vi "CAN Database Change Manager UI.vi"(8 "error in (no error)":errorcluster, 9 "VS Existing Frames":T1[](array[typedef]) {"Node Ref" format="%.0x"}, 10 "Old Cluster":refnum<k21>) -> (0 "error out":errorcluster, 2 "Cancel Out":bool, 3 "CAN Update":T4 {"Frames to Delete" format="%.0x"; "Frames to Update"."Node Ref" format="%.0x"})   [LabVIEW 2025, in "Protection and Counter Addon System Explorer.lvlib"]
uses:
  Protection and Counter Addon System Explorer.lvlib
  Types/CAN Update Results.ctl
  <vilib>/NI VeriStand/Custom Device API/Custom Device Item Ref.ctl
  Types/CAN Frame Update Results.ctl
  Types/CAN Filter Type.ctl
  Types/Base Frame Info_NoVS.ctl
  Types/Base Frame Info.ctl
  <vilib>/Utility/cursorutil.llb/Set Cursor (Icon Pict).vi
  <resource>/objmgr/xnet.rc
  <vilib>/NI VeriStand/Custom Device API/Custom Device API.lvlib
panel:
  in  "New Cluster":u16(ring)
  in  "New Database":refnum<k21>
  in  "Export":bool
  in  "Cancel":bool
  in  "Update":bool
  in  "Tree":string(tree)
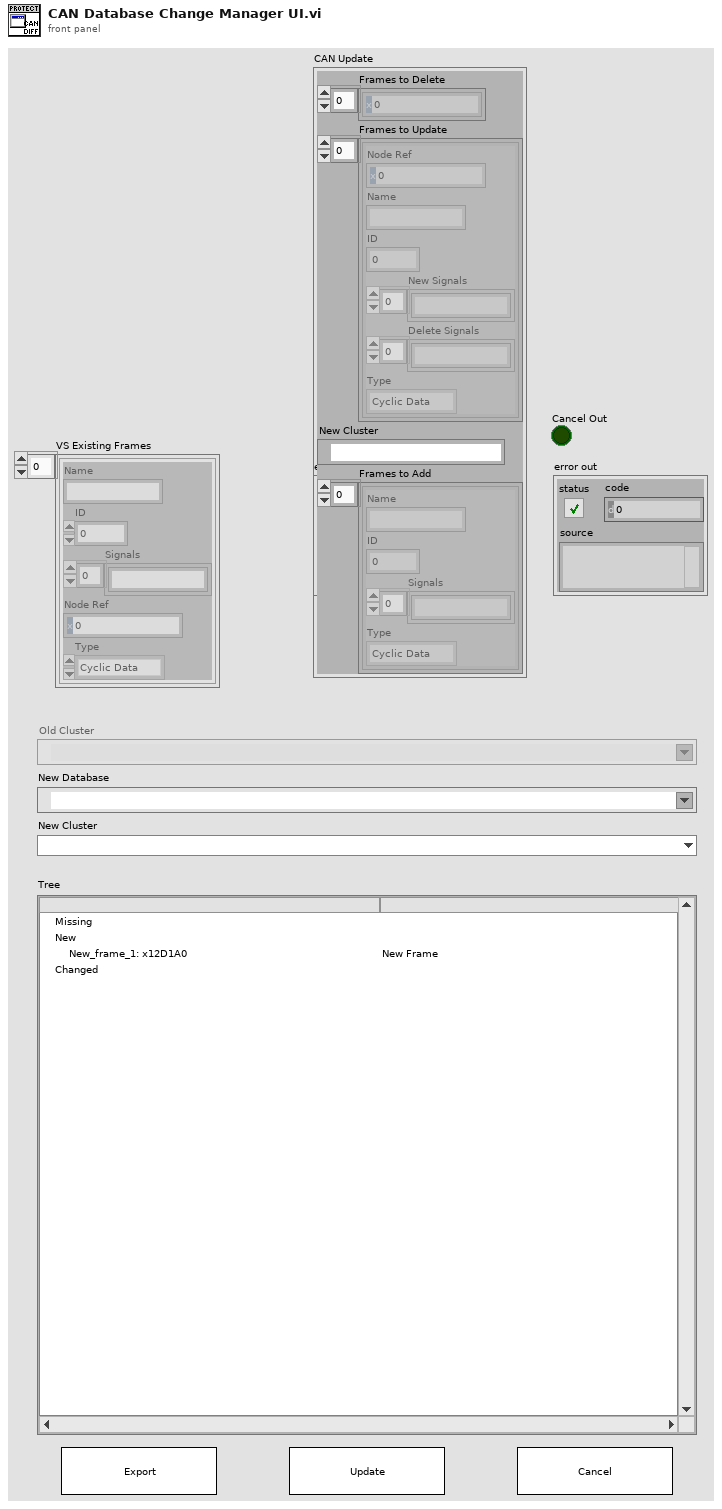
[diagram p1: front panel]
types:
  T1 = typedef "Protection and Counter Addon System Explorer.lvlib/Base Frame Info.ctl" = cluster{"Name":string, "ID":u32, "Signals":string[], "Node Ref":T2, "Type":T3}
  T2 = typedef "Custom Device API.lvlib/Custom Device Item Ref.ctl" = u64
  T3 = typedef "Protection and Counter Addon System Explorer.lvlib/CAN Filter Type.ctl" = enum16{"Cyclic Data", "Event Data", "Cyclic/Event", "All"}
  T4 = typedef "Protection and Counter Addon System Explorer.lvlib/CAN Update Results.ctl" = cluster{"Frames to Delete":T2[], "Frames to Update":T5[], "New Cluster":refnum<k21>, "Frames to Add":T6[]}
  T5 = typedef "Protection and Counter Addon System Explorer.lvlib/CAN Frame Update Results.ctl" = cluster{"Node Ref":T2, "Name":string, "ID":u32, "New Signals":string[], "Delete Signals":string[], "Type":T3}
  T6 = typedef "Protection and Counter Addon System Explorer.lvlib/Base Frame Info_NoVS.ctl" = cluster{"Name":string, "ID":u32, "Signals":string[], "Type":T3}
  T7 = enum8{"Enabled", "Disabled", "Disabled and Grayed Out"}
  T8 = typedef "Protection and Counter Addon System Explorer.lvlib/Database Changes.ctl" = cluster{"New":T6[], "Missing":T1[], "Changed":T9[]}
  T9 = typedef "Protection and Counter Addon System Explorer.lvlib/Related CAN Frames.ctl" = cluster{"Old":T1, "Change":T10}
  T10 = typedef "Protection and Counter Addon System Explorer.lvlib/Related CAN Frames No VS.ctl" = cluster{"New":T6, "Old":T6}
  T11 = typedef "LVPoint32TypeDef.ctl" = cluster{"Horizontal":i32, "Vertical":i32}
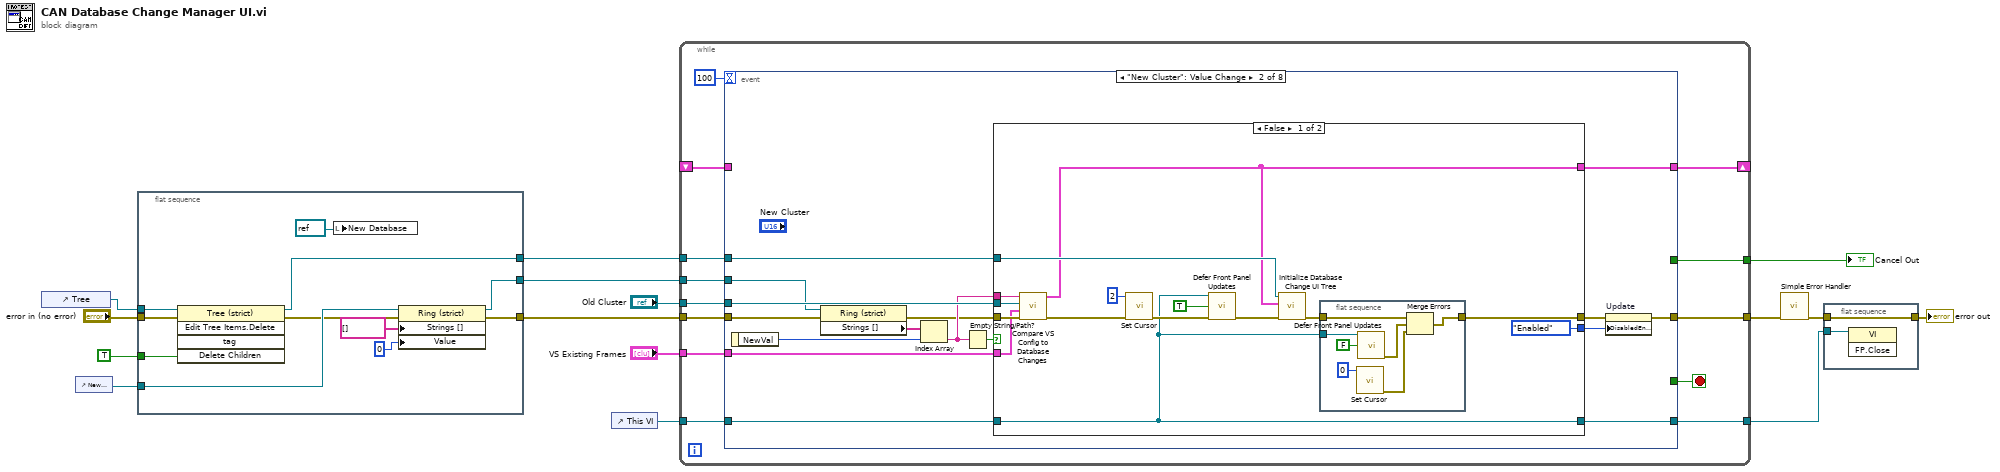
[diagram p0: block diagram]
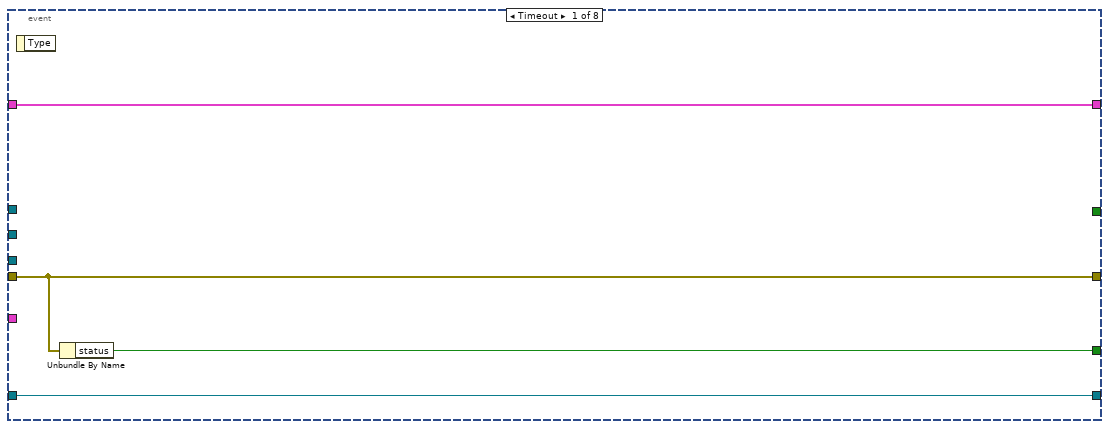
[diagram p2: hidden frame]
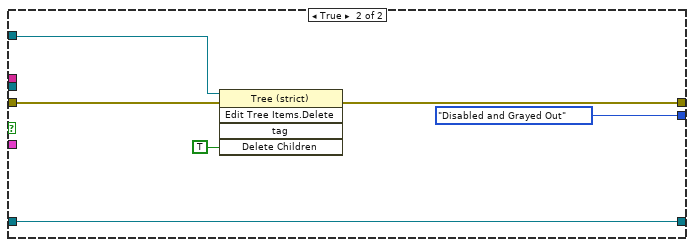
[diagram p3: hidden frame]
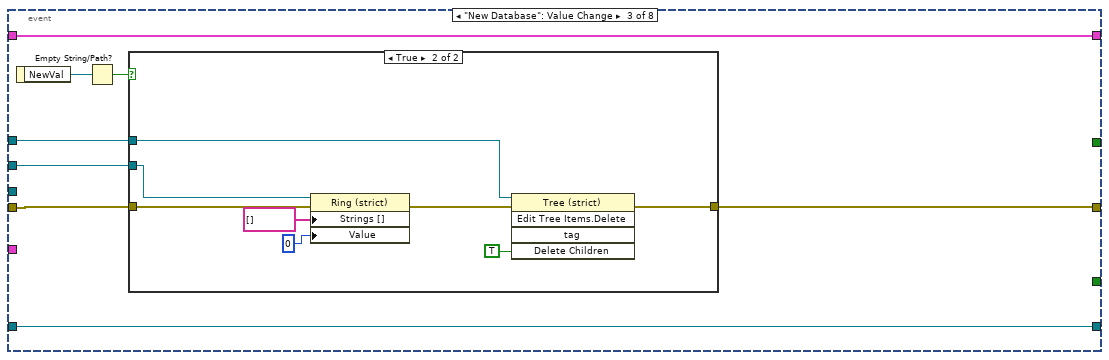
[diagram p4: hidden frame]
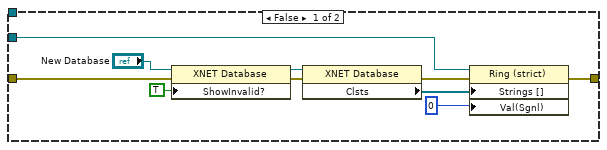
[diagram p5: hidden frame]
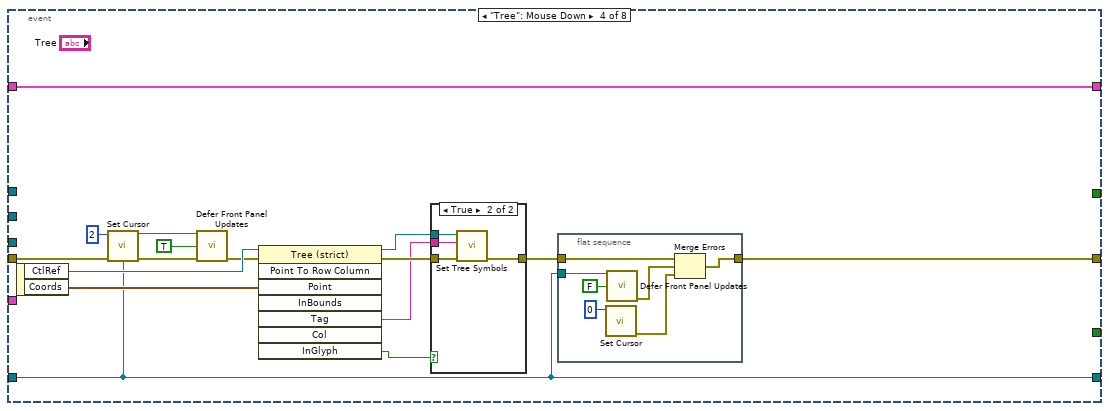
[diagram p6: hidden frame]
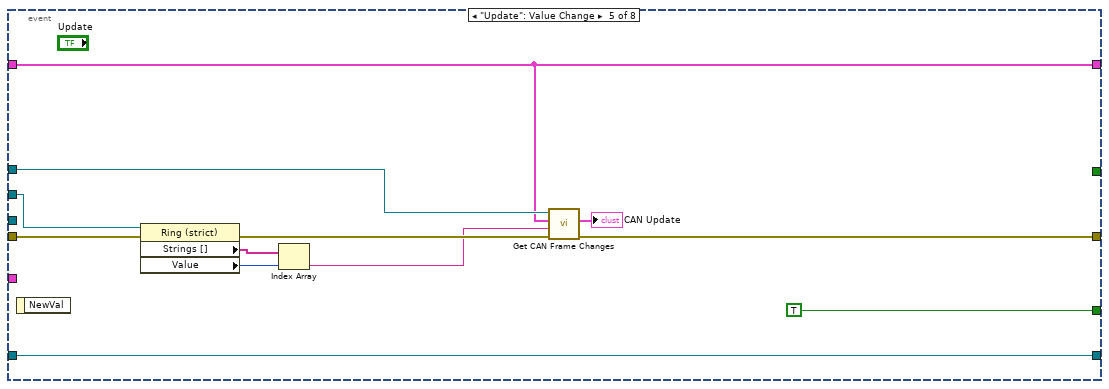
[diagram p8: hidden frame]
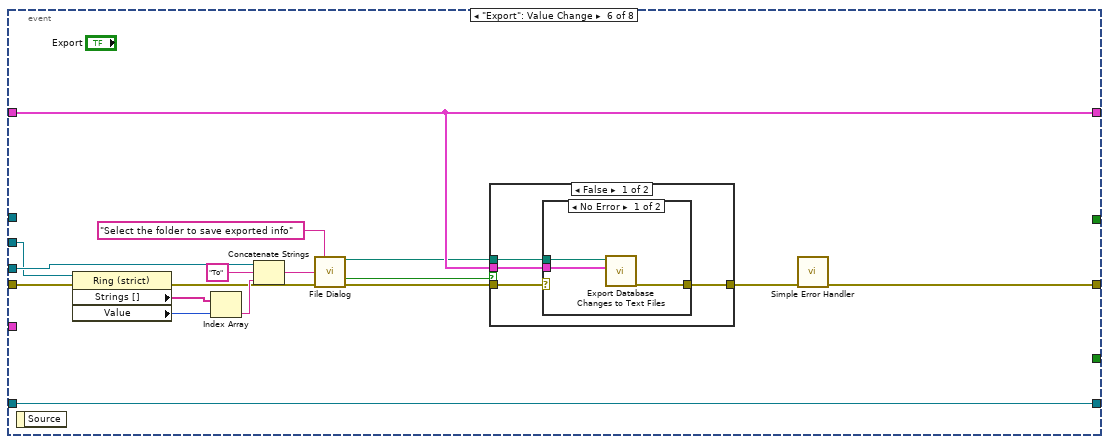
[diagram p9: hidden frame]
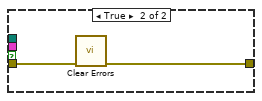
[diagram p11: hidden frame]
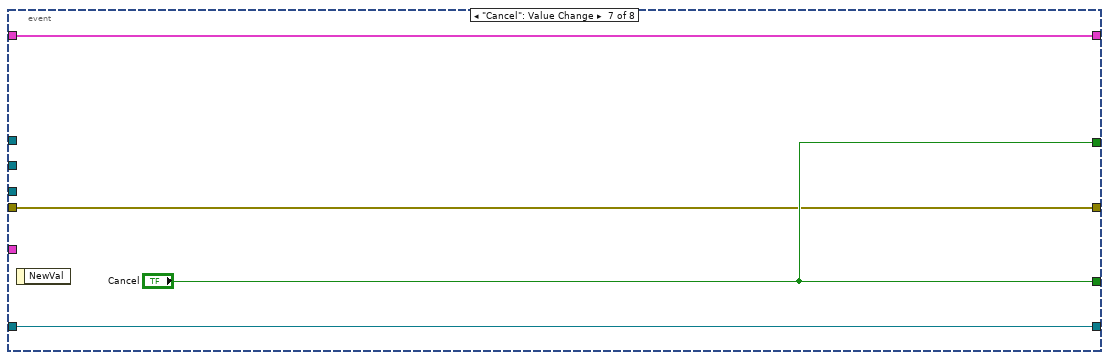
[diagram p12: hidden frame]
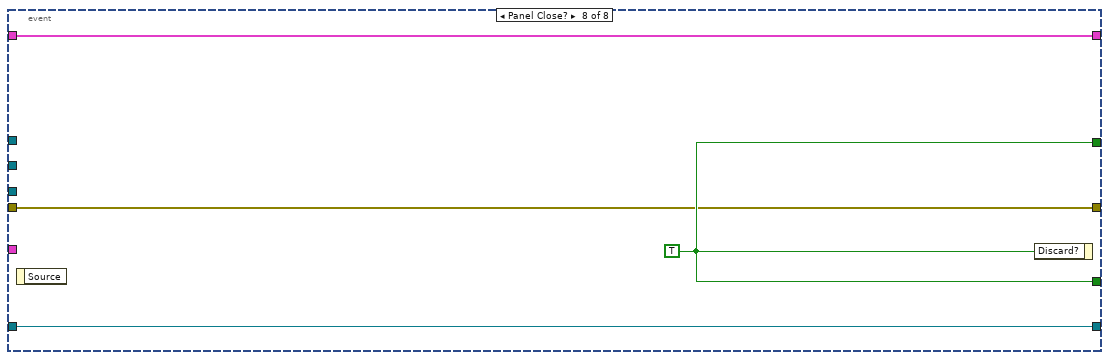
[diagram p13: hidden frame]
diagram:
  n1 = control-ref of="Tree"() -> (w6:refnum<vi>)
  n2 = control-ref of="New Cluster"() -> (w2:refnum<vi>)
  n3 = flat-sequence {
    tunnel: TRUE ("Delete Children?") -> [w26]
    tunnel: w6 -> [w25]
    tunnel: [w24] -> w5
    tunnel: "error in (no error)" -> [w23]
    tunnel: [w18] -> w3
    tunnel: w2 -> [w22]
    tunnel: [w17] -> w1
    frame #0 {
      n4 = invoke on="Invoke Node" class="Tree (strict)" method="Edit Tree Items.Delete"(reference=w25, error in=w23, "Delete Children"=w26) -> (reference out=w24:refnum<vi>, error out=w19:errorcluster)  [unwired: 2 in, 3 out]
      n5 = local write "New Database"(refnum<k21> refnum ("New Database")) -> ()
      n6 = property on="Property Node" class="Ring (strict)"(reference=w22, error in=w19, "Strings []"=string[] [], "Value"=u16 0) -> (reference out=w17:refnum<vi>, error out=w18:errorcluster)
    }
  }
  n7 = control-ref of="This VI"() -> (w9:refnum<vi>)
  n8 = while {
    tunnel: [w38] -> w14
    tunnel: [w37] -> w13
    tunnel: [w36] -> w12
    tunnel: "Old Cluster" -> [w34]
    tunnel: w5 -> [w33]
    tunnel: w9 -> [w32]
    tunnel: w3 -> [w31]
    shift-right: [w30] -> _
    shift-left: _ -> [w29]
    tunnel: "VS Existing Frames" -> [w28]
    tunnel: w1 -> [w27]
    stop <- w39 stop-if-true
    n9 = event shown="[1] \"New Cluster\": Value Change" {
      selector: _ -> [_ _ _ _ _ _ _ _]
      dyn-events: _ -> [_ _ _ _ _ _ _ _]
      timeout: 100 -> [_ _ _ _ _ _ _ _]
      tunnel: [w43 _ _ _ TRUE ("status") _ "Cancel" w187] -> w39
      tunnel: [w42 w52 w90 w120 w151 w163 w182 w186] -> w38
      tunnel: [w41 w55 w89 w116 w150 w169 w181 w185] -> w37
      tunnel: [_ _ _ _ _ _ "Cancel" w187] -> w36
      tunnel: w34 -> [_ w59 _ _ _ w162 _ _]
      tunnel: w33 -> [_ w58 w88 _ w149 _ _ _]
      tunnel: w32 -> [w41 w57 w89 w116 w150 w169 w181 w185]
      tunnel: w31 -> [w42 w45 w92 w115 w144 w156 w182 w186]
      tunnel: [w40 w56 w95 w114 w148 w168 w180 w184] -> w30
      tunnel: w29 -> [w40 _ w95 w114 w148 w168 w180 w184]
      tunnel: w28 -> [_ w50 _ _ _ _ _ _]
      tunnel: w27 -> [_ w44 w91 _ w146 w157 _ _]
      event Timeout {
        n10 = event-data() -> ()  [unwired: 1 in, 1 out]
        n11 = Unbundle By Name(w42) -> ("status"=w43:bool)
      }
      event "New Cluster": Value Change {
        n12 = event-data() -> ("NewVal"=w48:u16)  [unwired: 1 in]
        n13 = property class="Ring (strict)"(reference=w44, error in=w45) -> (error out=w46:errorcluster, "Strings []"=w49:string[])  [unwired: 1 out]
        n14 = Index Array(array=w49, index=w48) -> (element=w47:string)
        n15 = Empty String/Path?(string/path=w47) -> (empty?=w54:bool)
        n16 = case shown="False" w54 {
          tunnel: w59 -> [w71 _]
          tunnel: w47 -> [w70 _]
          tunnel: w58 -> [w69 w82]
          tunnel: w46 -> [w66 w83]
          tunnel: w57 -> [w63 w87]
          tunnel: [w64 w84] -> w53
          tunnel: [w60 _] -> w56
          tunnel: [w63 w87] -> w55
          tunnel: [T7."Enabled" ("Disabled") T7."Disabled and Grayed Out" ("Disabled")] -> w51
          tunnel: w50 -> [w61 _]
          frame False {
            n17 = call "Compare VS Config to Database Changes.vi"("error in (no error)"=w66, "VS Existing Frames"=w61, "Old Cluster"=w71, "New Cluster"=w70) -> ("error out"=w65:errorcluster, "Database Changes"=w60:T8)  [unwired: 6 in]
            n18 = call-poly <vilib>:"Set Cursor.vi"("error in (no error)"=w65, "icon"=u16 2) -> ("error out"=w72:errorcluster)  [unwired: 8 in, 1 out]
            n19 = call "Defer Front Panel Updates.vi"("This VI"=w63, "Defer Panel Updates"=TRUE, "error in (no error)"=w72) -> ("error out"=w73:errorcluster)  [unwired: 12 in]
            n20 = call "Initialize Database Change UI Tree.vi"("error in (no error)"=w73, "Database Changes"=w60, "TreeControl in"=w69) -> ("error out"=w74:errorcluster)  [unwired: 7 in, 1 out]
            n21 = flat-sequence {
              tunnel: [w80] -> w64
              tunnel: w74 -> [w79]
              tunnel: w63 -> [w77]
              frame #0 {
                n22 = call-poly <vilib>:"Set Cursor.vi"("icon"=u16 0) -> ("error out"=w75:errorcluster)  [unwired: 9 in, 1 out]
                n23 = call "Defer Front Panel Updates.vi"("This VI"=w77, "Defer Panel Updates"=FALSE) -> ("error out"=w78:errorcluster)  [unwired: 13 in]
                n24 = Merge Errors(w79, w78, w75) -> (w80:errorcluster)
              }
            }
          }
          frame True {
            n25 = invoke on="Invoke Node" class="Tree (strict)" method="Edit Tree Items.Delete"(reference=w82, error in=w83, "Delete Children"=TRUE ("Delete Children?")) -> (error out=w84:errorcluster)  [unwired: 2 in, 4 out]
          }
        }
        n26 = property on="Update" class="Bool"(error in=w53, "DisabledEnum"=w51) -> (error out=w52:errorcluster)  [unwired: 1 in, 1 out]
      }
      event "New Database": Value Change {
        n27 = event-data() -> ("NewVal"=w94:refnum<k21>)  [unwired: 1 in]
        n28 = Empty String/Path?(string/path=w94) -> (empty?=w93:bool)
        n29 = case shown="True" w93 {
          tunnel: w92 -> [w100 w106]
          tunnel: w91 -> [w98 w108]
          tunnel: [w96 w111] -> w90
          tunnel: w88 -> [_ w113]
          frame False {
            n30 = property class="XNET Database"(reference="New Database", error in=w100, "ShowInvalid?"=TRUE ("Show Invalid From Open?")) -> (reference out=w105:refnum<k21>, error out=w104:errorcluster)
            n31 = property class="XNET Database"(reference=w105, error in=w104) -> (error out=w97:errorcluster, "Clsts"=w101:refnum<k21>[])  [unwired: 1 out]
            n32 = property on="Property Node" class="Ring (strict)"(reference=w98, error in=w97, "Strings []"=w101, "Val(Sgnl)"=u16 0 ("Value (Signaling)")) -> (error out=w96:errorcluster)  [unwired: 1 out]
          }
          frame True {
            n33 = property on="Property Node" class="Ring (strict)"(reference=w108, error in=w106, "Strings []"=string[] [], "Value"=u16 0) -> (error out=w107:errorcluster)  [unwired: 1 out]
            n34 = invoke on="Invoke Node" class="Tree (strict)" method="Edit Tree Items.Delete"(reference=w113, error in=w107, "Delete Children"=TRUE ("Delete Children?")) -> (error out=w111:errorcluster)  [unwired: 2 in, 4 out]
          }
        }
      }
      event "Tree": Mouse Down {
        n35 = event-data() -> ("CtlRef"=w127:refnum<vi>, "Coords"=w128:T11)  [unwired: 1 in]
        n36 = call-poly <vilib>:"Set Cursor.vi"("error in (no error)"=w115, "icon"=u16 2) -> ("error out"=w118:errorcluster)  [unwired: 8 in, 1 out]
        n37 = call "Defer Front Panel Updates.vi"("This VI"=w116, "Defer Panel Updates"=TRUE, "error in (no error)"=w118) -> ("error out"=w117:errorcluster)  [unwired: 12 in]
        n38 = invoke on="Invoke Node" class="Tree (strict)" method="Point To Row Column"(reference=w127, error in=w117, "Point"=w128) -> (reference out=w125:refnum<vi>, error out=w126:errorcluster, "Tag"=w124:string, "InGlyph"=w123:bool)  [unwired: 5 in, 4 out]
        n39 = case shown="True" w123 {
          tunnel: w126 -> [w136 w140]
          tunnel: w125 -> [_ w139]
          tunnel: w124 -> [_ w138]
          tunnel: [w136 w137] -> w121
          frame False {
          }
          frame True {
            n40 = call "Set Tree Symbols.vi"("error in"=w140, "Tag"=w138, "CtlRef"=w139) -> ("error out"=w137:errorcluster)  [unwired: 8 in]
          }
        }
        n41 = flat-sequence {
          tunnel: [w132] -> w120
          tunnel: w121 -> [w133]
          tunnel: w116 -> [w129]
          frame #0 {
            n42 = call-poly <vilib>:"Set Cursor.vi"("icon"=u16 0) -> ("error out"=w134:errorcluster)  [unwired: 9 in, 1 out]
            n43 = call "Defer Front Panel Updates.vi"("This VI"=w129, "Defer Panel Updates"=FALSE) -> ("error out"=w130:errorcluster)  [unwired: 13 in]
            n44 = Merge Errors(w133, w130, w134) -> (w132:errorcluster)
          }
        }
      }
      event "Update": Value Change {
        n45 = event-data() -> ()  [unwired: 1 in, 1 out]
        n46 = property on="Property Node" class="Ring (strict)"(reference=w146, error in=w144) -> (error out=w145:errorcluster, "Strings []"=w143:string[], "Value"=w142:u16)  [unwired: 1 out]
        n47 = Index Array(array=w143, index=w142) -> (element=w141:string)
        n48 = call "Get CAN Frame Changes.vi"("error in (no error)"=w145, "New Cluster"=w141, "Database Changes"=w148, "TreeControl in"=w149) -> ("error out"=w151:errorcluster, "Change"=→"CAN Update":T4)  [unwired: 5 in, 1 out]
      }
      event "Export": Value Change {
        n49 = event-data() -> ()  [unwired: 1 in, 1 out]
        n50 = property on="Property Node" class="Ring (strict)"(reference=w157, error in=w156) -> (error out=w153:errorcluster, "Strings []"=w155:string[], "Value"=w158:u16)  [unwired: 1 out]
        n51 = Index Array(array=w155, index=w158) -> (element=w154:string)
        n52 = Concatenate Strings(w162, "To" ("string"), w154) -> (w160:string)
        n53 = call "File Dialog"("prompt"="Select the folder to save exported info", "default name"=w160, "error in"=w153) -> ("selected path"=w167:path, "cancelled"=w166:bool, "error out"=w165:errorcluster)  [unwired: 9 in, 1 out]
        n54 = case shown="False" w166 {
          tunnel: w168 -> [w173 _]
          tunnel: w167 -> [w172 _]
          tunnel: w165 -> [w170 w179]
          tunnel: [w171 w178] -> w164
          frame False {
            n55 = case shown="No Error" w170 {
              selector: w170 -> [_ w177]
              tunnel: w173 -> [w176 _]
              tunnel: w172 -> [w175 _]
              tunnel: [w174 w177] -> w171
              frame No Error {
                n56 = call "Export Database Changes to Text Files.vi"("Database Changes"=w176, "Folder"=w175) -> ("error out"=w174:errorcluster)  [unwired: 9 in]
              }
              frame Error {
              }
            }
          }
          frame True {
            n57 = call <vilib>:"Clear Errors.vi"("error in (no error)"=w179) -> ("error out"=w178:errorcluster)  [unwired: 5 in, 1 out]
          }
        }
        n58 = call <vilib>:"Simple Error Handler.vi"("error in (no error)"=w164) -> ("error out"=w163:errorcluster)  [unwired: 4 in, 4 out]
      }
      event "Cancel": Value Change {
        n59 = event-data() -> ()  [unwired: 1 in, 1 out]
      }
      event Panel Close? {
        w187 = TRUE ("Discard?")
        n60 = event-data() -> ()  [unwired: 1 in, 1 out]
        n61 = event-data("Discard?"=w187) -> ()  [unwired: 1 in, 1 out]
      }
    }
  }
  "Cancel Out" <- w12
  n62 = call <vilib>:"Simple Error Handler.vi"("error in (no error)"=w14) -> ("error out"=w15:errorcluster)  [unwired: 4 in, 4 out]
  n63 = flat-sequence {
    tunnel: [w189] -> w11
    tunnel: w15 -> [w189]
    tunnel: w13 -> [w188]
    frame #0 {
      n64 = invoke class="VI" method="FP.Close"(reference=w188) -> ()  [unwired: 2 in, 3 out]
    }
  }
  "error out" <- w11
